vi "Mapping Error Handler.vi"(8 "error in (no error)":errorcluster, 10 "Single Connect?":bool, 11 "Mapping Errors":T1[](array[typedef])) -> (0 "error out":errorcluster, 3 "Continue?":bool)   [LabVIEW 2016, in "System Mapping Tool.lvlib"]
uses:
  System Mapping Tool.lvlib
  TypeDefs/Mapping Error Cluster.ctl
  TypeDefs/Mapping Error.ctl
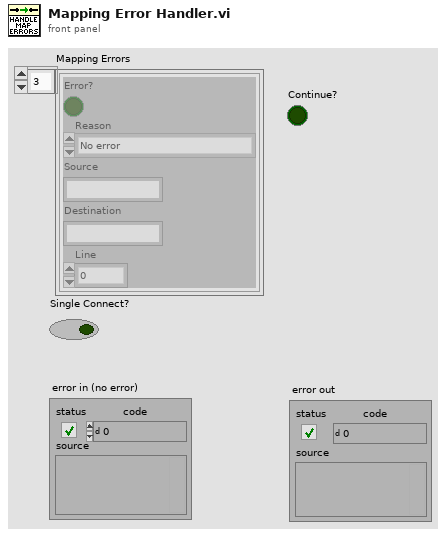
[diagram p1: front panel]
types:
  T1 = typedef "System Mapping Tool.lvlib/Mapping Error Cluster.ctl" = cluster{"Error?":bool, "Reason":T2, "Source":string, "Destination":string, "Line":i32}
  T2 = typedef "System Mapping Tool.lvlib/Mapping Error.ctl" = enum16{"No error", "Channels already mapped", "Source is not valid", "Destination is not valid", "Destination already mapped", "Destination mapped twice"}
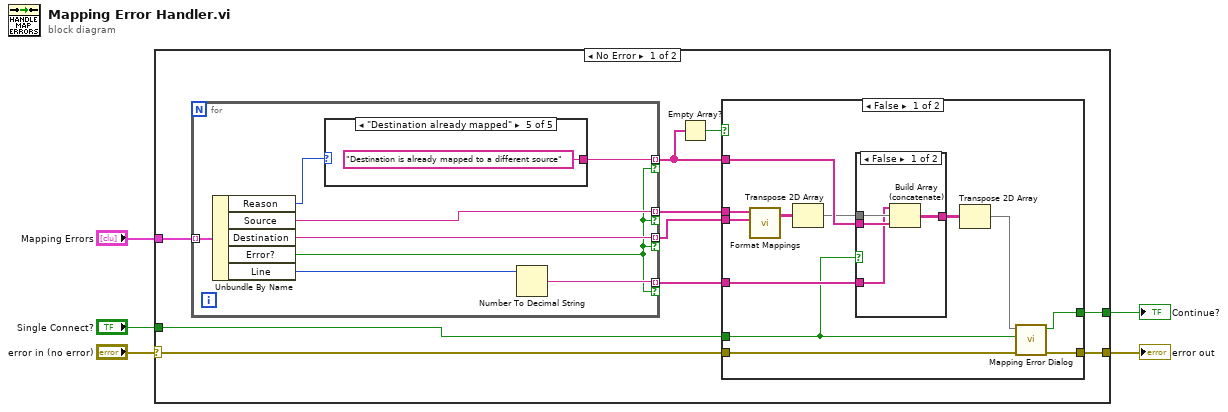
[diagram p0: block diagram]
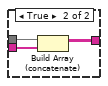
[diagram p2: hidden frame]
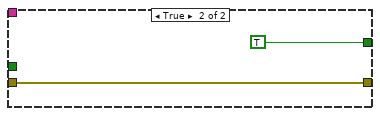
[diagram p3: hidden frame]
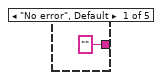
[diagram p4: hidden frame]
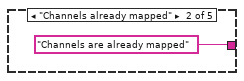
[diagram p5: hidden frame]
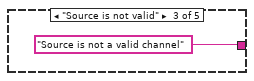
[diagram p6: hidden frame]
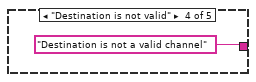
[diagram p7: hidden frame]
diagram:
  n1 = case shown="No Error" "error in (no error)" {
    selector: "error in (no error)" -> [w14 w50]
    tunnel: [w13 w50] -> w4
    tunnel: "Mapping Errors" -> [w15 _]
    tunnel: [w10 _] -> w2
    tunnel: "Single Connect?" -> [w7 _]
    frame No Error {
      n2 = for {
        tunnel: w15 -> [w44] mode=indexing
        tunnel: [w42] -> w11 mode=indexing if=w38
        tunnel: [w41] -> w12 mode=indexing if=w38
        tunnel: [w40] -> w9 mode=indexing if=w38
        tunnel: [w39] -> w6 mode=indexing if=w38
        n3 = Unbundle By Name(w44) -> ("Reason"=w43:T2, "Source"=w41:string, "Destination"=w42:string, "Error?"=w38:bool, "Line"=w37:i32)
        n4 = case shown="\"Destination already mapped\"" w43 {
          tunnel: ["" "Channels are already mapped" "Source is not a valid channel" "Destination is not a valid channel" "Destination is already mapped to a different source"] -> w40
          frame "No error", Default {
          }
          frame "Channels already mapped" {
          }
          frame "Source is not valid" {
          }
          frame "Destination is not valid" {
          }
          frame "Destination already mapped" {
          }
        }
        n5 = Number To Decimal String(number=w37) -> (decimal integer string=w39:string)  [unwired: 1 in]
      }
      n6 = Empty Array?(array=w9) -> (empty?=w8:bool)
      n7 = case shown="False" w8 {
        tunnel: w14 -> [w27 w36]
        tunnel: [w26 w36] -> w13
        tunnel: w12 -> [w25 _]
        tunnel: w11 -> [w24 _]
        tunnel: w9 -> [w22 _]
        tunnel: [w18 TRUE ("Continue?")] -> w10
        tunnel: w7 -> [w16 _]
        tunnel: w6 -> [w17 _]
        frame False {
          n8 = call "Format Mappings.vi"("Destinations"=w24, "Sources"=w25) -> ("Mappings"=w23:string[][])  [unwired: 3 in]
          n9 = Transpose 2D Array(2D array=w23) -> (transposed array=w20:string[][])
          n10 = case shown="False" w16 {
            tunnel: w22 -> [w31 w33]
            tunnel: [w30 w32] -> w21
            tunnel: w20 -> [w29 w34]
            tunnel: w17 -> [w28 _]
            frame False {
              n11 = Build Array (concatenate)(w28, w29, w31) -> (w30:string[][])
            }
            frame True {
              n12 = Build Array (concatenate)(w34, w33) -> (w32:string[][])
            }
          }
          n13 = Transpose 2D Array(2D array=w21) -> (transposed array=w19:string[][])
          n14 = call "Mapping Error Dialog.vi"("error in (no error)"=w27, "Single Connect?"=w16, "Mapping Errors"=w19) -> ("error out"=w26:errorcluster, "Continue?"=w18:bool)  [unwired: 7 in]
        }
        frame True {
        }
      }
    }
    frame Error {
    }
  }
  "error out" <- w4
  "Continue?" <- w2
